vi "Sensor_Values.vi"() -> ()   [LabVIEW 2020]
panel:
  out "Limelight_Disconnected":bool
  in  "Turret_Absolute_Position(Degrees)":dbl=0.00775835173077931
  out "Safe_To_Move_Turret?":bool
  in  "Outer_Arm_Elevator_Position(inches)":dbl
  in  "Magazine_Velocity(ticks/100ms)":dbl(graph)
  out "Ball_In_Funnel":bool
  out "Limelight_Has_Target?":bool
  in  "Drive_IMU_Pitch (deg)":dbl=0.791015625
  in  "Cowl_Angle(deg)":dbl=61.6
  in  "Limelight_Distance_To_Target (in)":dbl=89.24378251445923
  in  "Camera_Goal_Y (deg)":dbl
  out "Magazine_Loaded":bool
  in  "Outer_Arm_Elevator_Position (ticks)":i32
  in  "Safe_Module_Latch_Angle(deg)":dbl
  in  "Pose_Loop_Time(ms)":u32=29
  in  "Robot_Ground_Speed(ft/s)":dbl
  in  "Robot_Y_Position(in)":dbl=0.006777704740323944
  in  "Robot_X_Position(in)":dbl=-0.0006721278033652426
  in  "Flywheel_Velocity(RPM)":dbl
  in  "Camera_Goal_X (deg)":dbl
  in  "Flywheel_Right_Velocity":dbl
  in  "Flywheel_Left_Velocity":dbl
  in  "Turret_Relative_Position(Degrees)":dbl=0.00775835173077931
  in  "Camera_X_Offset":dbl
  in  "Camera_Area":dbl
  in  "Drive_IMU_Yaw (deg)":dbl=271.20574951171875
  in  "Back_Right_Wheel_Angle (deg)":dbl=-177.007421875
  in  "Back_Left_Wheel_Angle (deg)":dbl=3.433437500000025
  in  "Front_Left_Wheel_Angle (deg)":dbl=5.0146874999999795
  in  "Front_Right_Wheel_Angle (deg)":dbl=2.554374999999993
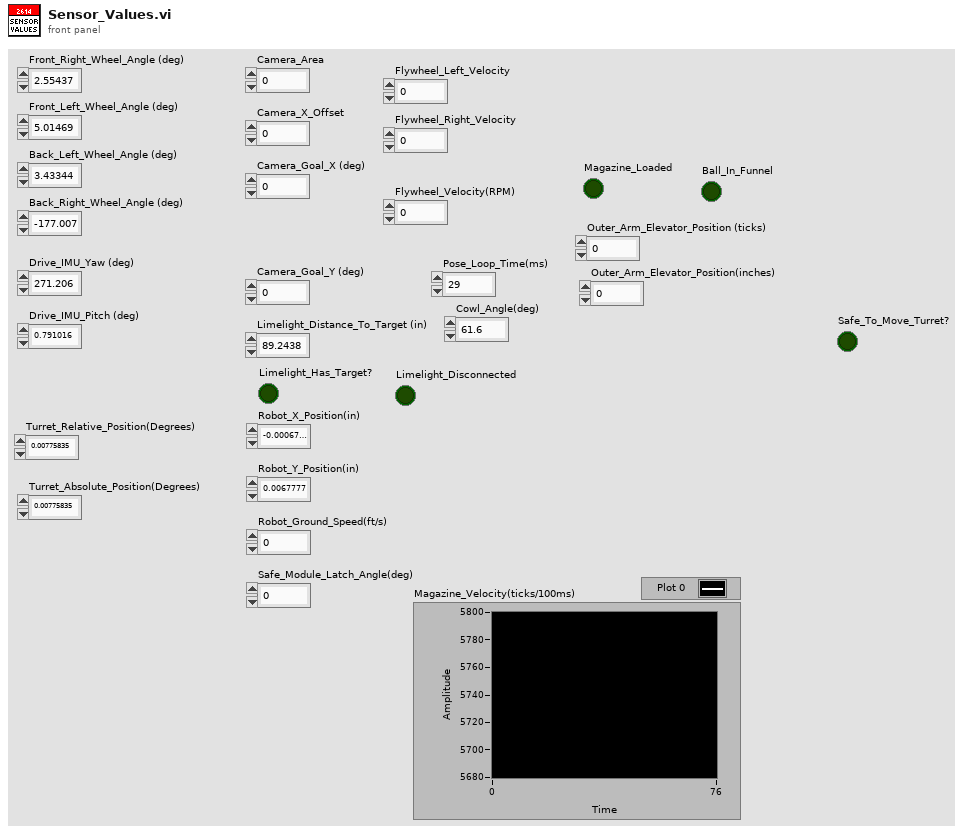
[diagram p1: front panel]
diagram:
